vi "总磷总氮量程读取.vi"(8 "error in (no error)":errorcluster caption="错误输入（无错误）", 9 "量程":enum16{"低量程", "高量程"}(ring), 10 "测量模式":enum16{"水样测量", "零点核查", "跨度核查", "标样核查", "加标回收"}(ring), 11 "测量参数":enum16{"总磷", "总氮"}(ring)) -> (0 "error out":errorcluster caption="错误输出", 3 "量程切换阈值":cluster{"阈值":dbl, "标液浓度":dbl})   [LabVIEW 2016, in "斯坦道总磷总氮.lvlib"]
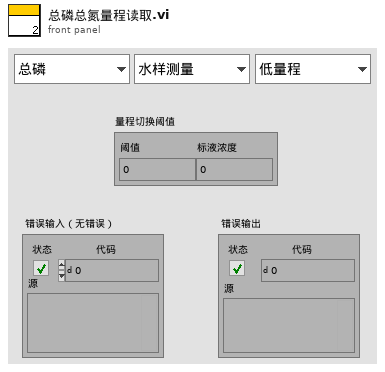
[diagram p1: front panel]
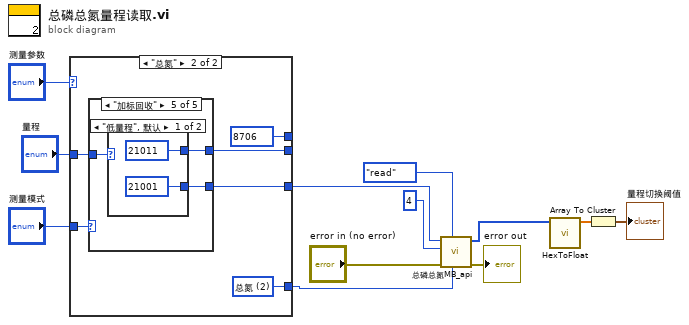
[diagram p0: block diagram]
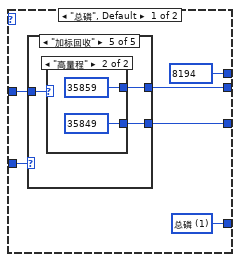
[diagram p2: hidden frame]
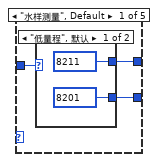
[diagram p3: hidden frame]
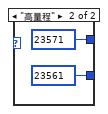
[diagram p4: hidden frame]
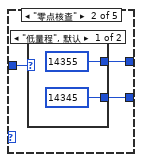
[diagram p5: hidden frame]
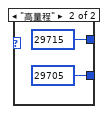
[diagram p6: hidden frame]
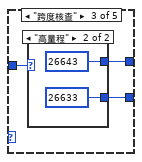
[diagram p7: hidden frame]
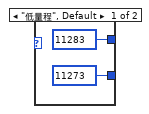
[diagram p8: hidden frame]
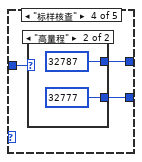
[diagram p9: hidden frame]
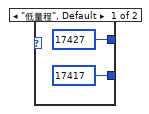
[diagram p10: hidden frame]
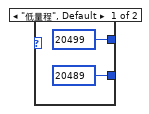
[diagram p11: hidden frame]
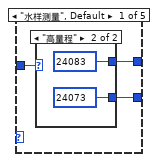
[diagram p12: hidden frame]
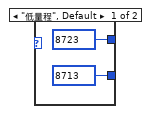
[diagram p13: hidden frame]
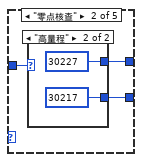
[diagram p14: hidden frame]
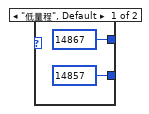
[diagram p15: hidden frame]
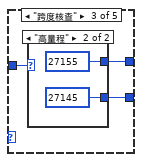
[diagram p16: hidden frame]
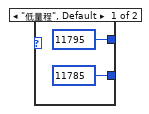
[diagram p17: hidden frame]
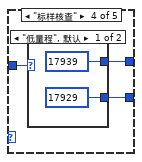
[diagram p18: hidden frame]
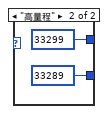
[diagram p19: hidden frame]
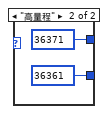
[diagram p20: hidden frame]
diagram:
  n1 = case shown="\"总氮\"" "测量参数" {
    tunnel: "测量模式" -> [w18 w56]
    tunnel: "量程" -> [w17 w57]
    tunnel: [w16 w59] -> w2
    tunnel: [w15 w54] -> _
    tunnel: [w14 w55] -> w9
    tunnel: [u16 8194 ("starting address") u16 8706 ("starting address")] -> _
    frame "总磷", Default {
      w16 = u16 1 items=["总磷"=1, "氨氮"=3] ("站号")
      n2 = case shown="\"加标回收\"" w18 {
        tunnel: w17 -> [w21 w28 w35 w42 w49]
        tunnel: [w20 w27 w34 w41 w48] -> w15
        tunnel: [w19 w26 w33 w40 w47] -> w14
        frame "水样测量", Default {
          n3 = case shown="\"低量程\", 默认" w21 {
            tunnel: [u16 8211 ("starting address") u16 23571 ("starting address")] -> w20
            tunnel: [u16 8201 ("starting address") u16 23561 ("starting address")] -> w19
            frame "低量程", Default {
            }
            frame "高量程" {
            }
          }
        }
        frame "零点核查" {
          n4 = case shown="\"低量程\", 默认" w28 {
            tunnel: [u16 14355 ("starting address") u16 29715 ("starting address")] -> w27
            tunnel: [u16 14345 ("starting address") u16 29705 ("starting address")] -> w26
            frame "低量程", Default {
            }
            frame "高量程" {
            }
          }
        }
        frame "跨度核查" {
          n5 = case shown="\"高量程\"" w35 {
            tunnel: [u16 11283 ("starting address") u16 26643 ("starting address")] -> w34
            tunnel: [u16 11273 ("starting address") u16 26633 ("starting address")] -> w33
            frame "低量程", Default {
            }
            frame "高量程" {
            }
          }
        }
        frame "标样核查" {
          n6 = case shown="\"高量程\"" w42 {
            tunnel: [u16 17427 ("starting address") u16 32787 ("starting address")] -> w41
            tunnel: [u16 17417 ("starting address") u16 32777 ("starting address")] -> w40
            frame "低量程", Default {
            }
            frame "高量程" {
            }
          }
        }
        frame "加标回收" {
          n7 = case shown="\"高量程\"" w49 {
            tunnel: [u16 20499 ("starting address") u16 35859 ("starting address")] -> w48
            tunnel: [u16 20489 ("starting address") u16 35849 ("starting address")] -> w47
            frame "低量程", Default {
            }
            frame "高量程" {
            }
          }
        }
      }
    }
    frame "总氮" {
      w59 = u16 2 items=["总磷"=1, "总氮"=2, "氨氮"=3] ("站号")
      n8 = case shown="\"加标回收\"" w56 {
        tunnel: w57 -> [w62 w69 w76 w83 w90]
        tunnel: [w61 w68 w75 w82 w89] -> w54
        tunnel: [w60 w67 w74 w81 w88] -> w55
        frame "水样测量", Default {
          n9 = case shown="\"高量程\"" w62 {
            tunnel: [u16 8723 ("starting address") u16 24083 ("starting address")] -> w61
            tunnel: [u16 8713 ("starting address") u16 24073 ("starting address")] -> w60
            frame "低量程", Default {
            }
            frame "高量程" {
            }
          }
        }
        frame "零点核查" {
          n10 = case shown="\"高量程\"" w69 {
            tunnel: [u16 14867 ("starting address") u16 30227 ("starting address")] -> w68
            tunnel: [u16 14857 ("starting address") u16 30217 ("starting address")] -> w67
            frame "低量程", Default {
            }
            frame "高量程" {
            }
          }
        }
        frame "跨度核查" {
          n11 = case shown="\"高量程\"" w76 {
            tunnel: [u16 11795 ("starting address") u16 27155 ("starting address")] -> w75
            tunnel: [u16 11785 ("starting address") u16 27145 ("starting address")] -> w74
            frame "低量程", Default {
            }
            frame "高量程" {
            }
          }
        }
        frame "标样核查" {
          n12 = case shown="\"低量程\", 默认" w83 {
            tunnel: [u16 17939 ("starting address") u16 33299 ("starting address")] -> w82
            tunnel: [u16 17929 ("starting address") u16 33289 ("starting address")] -> w81
            frame "低量程", Default {
            }
            frame "高量程" {
            }
          }
        }
        frame "加标回收" {
          n13 = case shown="\"低量程\", 默认" w90 {
            tunnel: [u16 21011 ("starting address") u16 36371 ("starting address")] -> w89
            tunnel: [u16 21001 ("starting address") u16 36361 ("starting address")] -> w88
            frame "低量程", Default {
            }
            frame "高量程" {
            }
          }
        }
      }
    }
  }
  n14 = call "总磷总氮MB_api.vi"("Slave ID"=w2, "STEP"=enum16{"open", "read", "write", "close"}."read", "Error in"="error in (no error)", "quantity"=u16 4, "starting address"=w9) -> ("error out"=→"error out":errorcluster, "Registers"=w5:u16[])  [unwired: 4 in, 1 out]
  n15 = call "HexToFloat.vi"("数组"=w5) -> ("FLOAT"=w4:sgl[])  [unwired: 10 in]
  n16 = Array To Cluster(array=w4) -> (cluster=→"量程切换阈值":cluster{"FLOAT[0]":sgl, "FLOAT[1]":sgl})
